vi "pattern_recognition.vi"(0 "read buffer in":string) -> (2 "read buffer out":string, 3 "Boolean":bool)   [LabVIEW 2018]
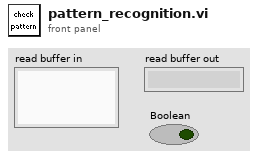
[diagram p1: front panel]
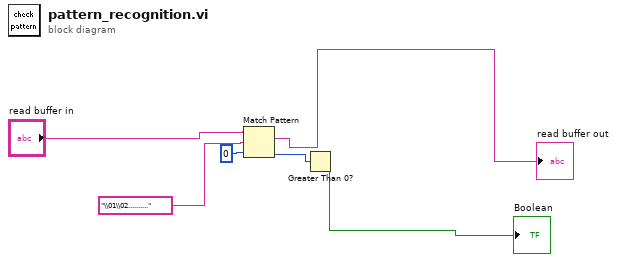
[diagram p0: block diagram]
diagram:
  n1 = Match Pattern(string="read buffer in", regular expression="\\01\\02..........", offset (0)=0) -> (match substring=→"read buffer out":string, offset past match=w2:i32)  [unwired: 2 out]
  n2 = Greater Than 0?(x=w2) -> (x > 0?=→"Boolean":bool)
